vi "philosopher_regex.vi"(5 "Maximum attempts":i32, 6 "Maximum think time":u32=1000, 7 "Maximum eat time":u32=1000, 9 "Dummy":i32, 10 "Ph id":i32) -> ()   [LabVIEW 2015]
uses:
  SINGLE_CHOP_Separator_string.ctl
panel:
  out "keys":string[](array[string])
  # "Viene LANCIATO DA PHILOSOFERS"
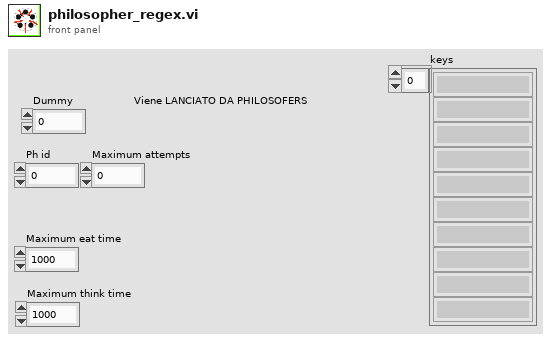
[diagram p1: front panel]
types:
  T1 = typedef "SINGLE_CHOP_Separator_string.ctl" = string
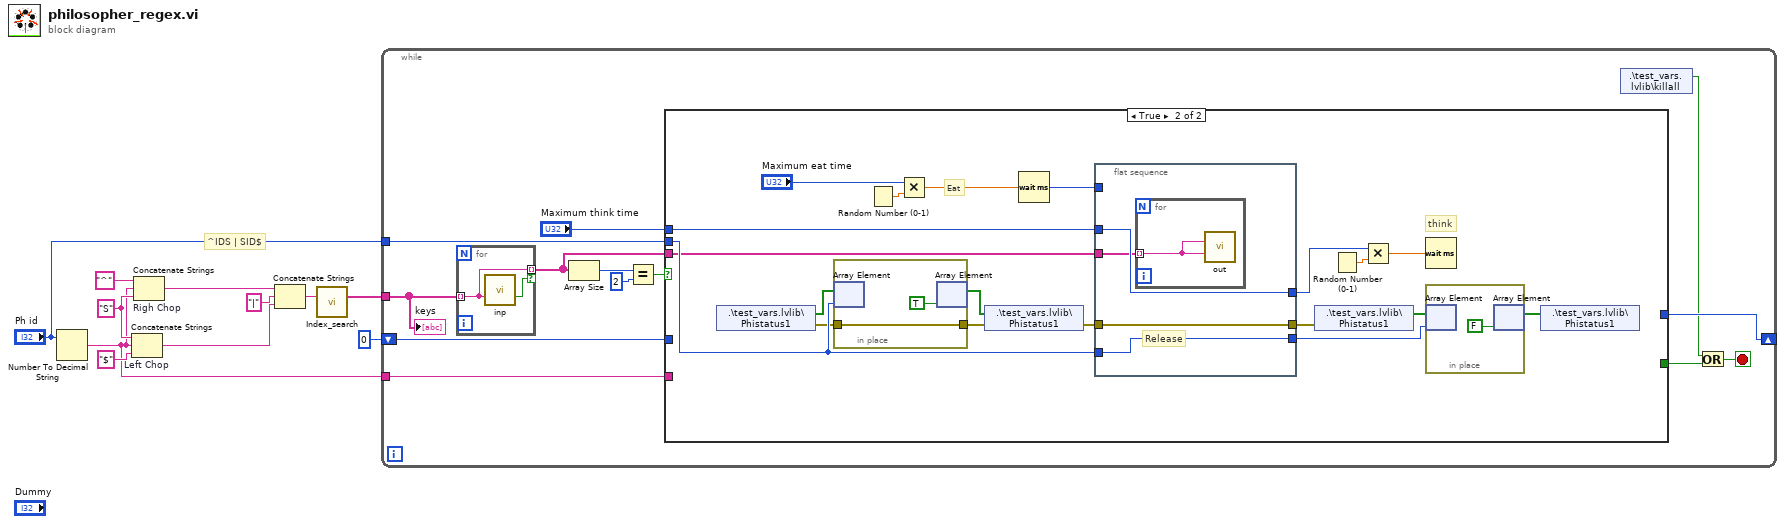
[diagram p0: block diagram]
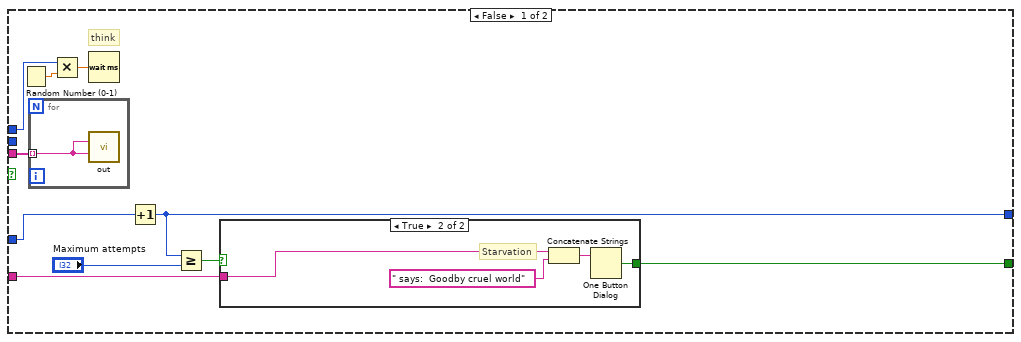
[diagram p2: hidden frame]
diagram:
  w4 = T1 "S"
  # "^IDS | SID$"
  n1 = Number To Decimal String(number="Ph id") -> (decimal integer string=w3:string)  [unwired: 1 in]
  n2 = Concatenate Strings "Left Chop"(w4, w3, "$" ("string")) -> (w8:string)
  n3 = Concatenate Strings "Righ Chop"("^" ("string"), w3, w4) -> (w9:string)
  n4 = Concatenate Strings(w9, "|" ("string"), w8) -> (w2:string)
  n5 = call "Index_search.vi"("Regex"=w2) -> ("keys"=w1:string[])  [unwired: 7 in, 7 out]
  n6 = while {
    shift-right: [w23] -> _
    shift-left: 0 -> [w24]
    tunnel: "Ph id" -> [w18]
    tunnel: w3 -> [w17]
    tunnel: w1 -> [w12]
    stop <- w20 stop-if-true
    n7 = for {
      tunnel: w12 -> [w26] mode=indexing
      tunnel: [w26] -> w13 mode=indexing if=w25
      n8 = call "inp.vi"("Name in"=w26) -> ("Valid data"=w25:bool)  [unwired: 12 in, 2 out]
    }
    n9 = Array Size(array=w13) -> (size(s)=w16:i32)
    n10 = Equal?(x=w16, y=2) -> (x = y?=w14:bool)
    n11 = case shown="True" w14 {
      tunnel: w24 -> [w36 _]
      tunnel: [w33 _] -> w19
      tunnel: [w32 _] -> w23
      tunnel: w17 -> [w29 _]
      tunnel: "Maximum think time" -> [w28 w54]
      tunnel: w18 -> [_ w47]
      tunnel: w13 -> [w27 w42]
      frame False {
        # "think"
        n12 = Random Number (0-1)() -> (number: 0 to 1=w31:dbl)
        n13 = for {
          tunnel: w27 -> [w37] mode=indexing
          n14 = call "out.vi"("IN VARIANT"=w37, "Name in"=w37) -> ()  [unwired: 12 in, 2 out]
        }
        n15 = Multiply(x=w28, y=w31) -> (x*y=w30:dbl)
        n16 = Wait (ms)(milliseconds to wait=w30) -> ()  [unwired: 1 out]
        n17 = Increment(x=w36) -> (x+1=w32:i32)
        n18 = Greater Or Equal?(x=w32, y="Maximum attempts") -> (x >= y?=w34:bool)
        n19 = case shown="True" w34 {
          tunnel: [_ w41] -> w33
          tunnel: w29 -> [_ w40]
          frame False {
          }
          frame True {
            # "Starvation"
            n20 = Concatenate Strings(w40, " says:  Goodby cruel world" ("message")) -> (w38:string)
            n21 = One Button Dialog(message=w38) -> (true=w41:bool)  [unwired: 1 in]
          }
        }
      }
      frame True {
        # "think"
        # "Eat"
        n22 = shared-variable ".\\test_vars.lvlib\\Phistatus1"() -> (w52:bool[], error out=w45:errorcluster)  [unwired: 1 in]
        n23 = in-place {
          in-place-border: w45 -> [w62]
          in-place-border: [w62] -> w44
          n24 = in-place-array #1(w52, w47) -> ()  [unwired: 1 out]
          n25 = in-place-array #1(TRUE ("element")) -> (w51:bool[])  [unwired: 1 out]
        }
        n26 = Random Number (0-1)() -> (number: 0 to 1=w59:dbl)
        n27 = Multiply(x="Maximum eat time", y=w59) -> (x*y=w57:dbl)
        n28 = shared-variable ".\\test_vars.lvlib\\Phistatus1"(w51, error in=w44) -> (error out=w50:errorcluster)
        n29 = Wait (ms)(milliseconds to wait=w57) -> (millisecond timer value=w60:u32)
        n30 = flat-sequence {
          tunnel: w60 -> [_]
          tunnel: [w67] -> w53
          tunnel: w54 -> [w67]
          tunnel: w50 -> [w65]
          tunnel: [w66] -> w46
          tunnel: w47 -> [w66]
          tunnel: [w65] -> w43
          tunnel: w42 -> [w64]
          frame #0 {
            # "Release"
            n31 = for {
              tunnel: w64 -> [w68] mode=indexing
              n32 = call "out.vi"("IN VARIANT"=w68, "Name in"=w68) -> ()  [unwired: 12 in, 2 out]
            }
          }
        }
        n33 = shared-variable ".\\test_vars.lvlib\\Phistatus1"(error in=w43) -> (w48:bool[])  [unwired: 1 out]
        n34 = Random Number (0-1)() -> (number: 0 to 1=w56:dbl)
        n35 = Multiply(x=w53, y=w56) -> (x*y=w55:dbl)
        n36 = Wait (ms)(milliseconds to wait=w55) -> ()  [unwired: 1 out]
        n37 = in-place {
          n38 = in-place-array #2(w48, w46) -> ()  [unwired: 1 out]
          n39 = in-place-array #2(FALSE ("element")) -> (w49:bool[])  [unwired: 1 out]
        }
        n40 = shared-variable ".\\test_vars.lvlib\\Phistatus1"(w49) -> ()  [unwired: 1 in, 1 out]
      }
    }
    n41 = shared-variable ".\\test_vars.lvlib\\killall"() -> (w21:bool)  [unwired: 1 in, 1 out]
    n42 = Or(x=w21, y=w19) -> (x .or. y?=w20:bool)
    "keys" <- w12
  }
